vi "Measurement-DC.vi"(6 "引用句柄输出":refnum<file>, 7 "Ctl Refnum":refnum<vi>, 8 "error in (no error)":errorcluster caption="错误输入（无错误）", 9 "升温速率":dbl, 10 "结束温度":dbl, 11 "簇":T1) -> (0 "error out":errorcluster caption="错误输出", 1 "极化电流":dbl, 2 "布尔":bool, 3 "当前温度":dbl)   [LabVIEW 2017]
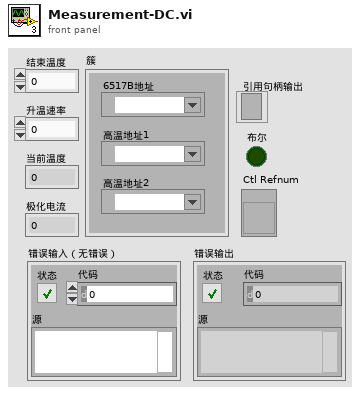
[diagram p1: front panel]
types:
  T1 = cluster{"6517B地址":refnum<visa-resource-name>, "高温地址1":refnum<visa-resource-name>, "高温地址2":refnum<visa-resource-name>}
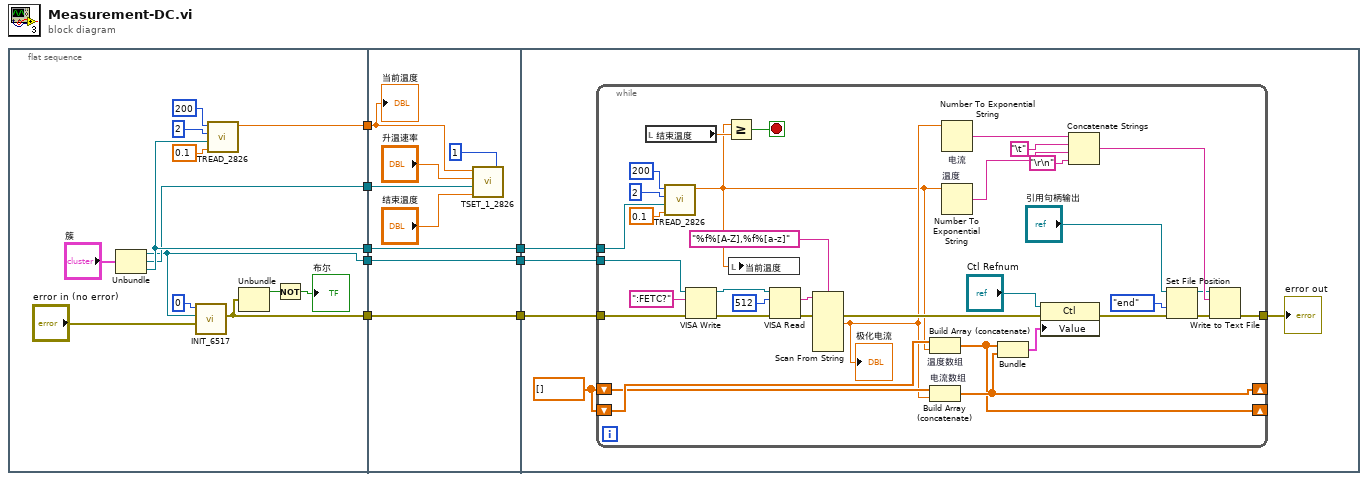
[diagram p0: block diagram]
diagram:
  n1 = flat-sequence {
    tunnel: [w17] -> w8
    tunnel: [w15] -> w6
    tunnel: [w14] -> w5
    tunnel: [w12] -> w3
    tunnel: [w11] -> w1
    tunnel: w8 -> [w29]
    tunnel: [w29] -> w7
    tunnel: w6 -> [w28]
    tunnel: w5 -> [w26]
    tunnel: [w23] -> w4
    tunnel: w3 -> [w23]
    tunnel: [w22] -> w2
    tunnel: w1 -> [w22]
    tunnel: w7 -> [w34]
    tunnel: w4 -> [w33]
    tunnel: w2 -> [w32]
    frame #0 {
      n2 = Unbundle("簇") -> ("6517B地址"=w12:refnum<visa-resource-name>, "高温地址1"=w15:refnum<visa-resource-name>, "高温地址2"=w17:refnum<visa-resource-name>)
      n3 = call "INIT_6517.vi"("error in (no error)"="error in (no error)", "VISA resource name"=w12, "Vin"=0) -> ("error out"=w11:errorcluster)  [unwired: 7 in, 1 out]
      n4 = call "TREAD_2826.vi"("Unknown Param 2"=0.1, "VISA resource name"=w17, "Address No."=2, "Unknown Param"=200) -> ("PV"=w14:dbl)  [unwired: 3 out]
      n5 = Unbundle(w11) -> ("status"=w9:bool)  [unwired: 2 out]
      n6 = Not(x=w9) -> (.not. x?=→"布尔":bool)
    }
    frame #1 {
      n7 = call "TSET_1_2826.vi"("Address No."=1, "T-Ending, C"="结束温度", "VISA resource name"=w28, "cooling/heating rate, C/min"="升温速率", "T-Starting, C"=w26) -> ()
      "当前温度" <- w26
    }
    frame #2 {
      w31 = dbl[] []
      n8 = while {
        tunnel: w34 -> [w69]
        tunnel: w33 -> [w62]
        tunnel: w32 -> [w61]
        shift-right: [w51] -> _
        shift-left: w31 -> [w54]
        shift-right: [w52] -> _
        shift-left: w31 -> [w53]
        tunnel: [w46] -> w30
        stop <- w64 stop-if-true
        n9 = local read "结束温度"() -> (w65:dbl)
        n10 = call "TREAD_2826.vi"("Unknown Param 2"=0.1, "VISA resource name"=w69, "Address No."=2, "Unknown Param"=200) -> ("PV"=w35:dbl)  [unwired: 3 out]
        n11 = VISA Write(VISA resource name=w62, write buffer=":FETC?" ("写入缓冲区"), error in (no error)=w61) -> (VISA resource name out=w58:refnum<visa-resource-name>, error out=w60:errorcluster)  [unwired: 1 out]
        n12 = Greater Or Equal?(x=w35, y=w65) -> (x >= y?=w64:bool)
        n13 = local write "当前温度"(w35) -> ()
        n14 = VISA Read(VISA resource name=w58, byte count=u32 512 ("字节总数"), error in (no error)=w60) -> (read buffer=w57:string, error out=w56:errorcluster)  [unwired: 2 out]
        n15 = Scan From String(format string="%f%[A-Z],%f%[a-z]" ("格式字符串"), input string=w57, error in=w56) -> (error out=w48:errorcluster, output 1=w36:dbl)  [unwired: 1 in, 9 out]
        "极化电流" <- w36
        n16 = Build Array (concatenate) "温度数组"(w54, w35) -> (w51:dbl[])
        n17 = Build Array (concatenate) "电流数组"(w53, w36) -> (w52:dbl[])
        n18 = Number To Exponential String "电流"(number=w36) -> (E-format string=w43:string)  [unwired: 1 in, 2 out]
        n19 = Number To Exponential String "温度"(number=w35) -> (E-format string=w42:string)  [unwired: 3 out]
        n20 = Bundle(w51, w52) -> (w49:cluster{dbl[], dbl[]})  [unwired: 1 in]
        n21 = property class="Ctl"(reference="Ctl Refnum", error in=w48, "Value"=w49) -> (error out=w45:errorcluster)  [unwired: 1 out]
        n22 = Concatenate Strings(w43, "\t", w42, "\r\n") -> (w39:string)
        n23 = Set File Position(refnum="引用句柄输出", from (0:start)=enum16{"start", "end", "current"}."end" ("自（0:起始）"), error in=w45) -> (refnum out=w38:refnum<file>, error out=w47:errorcluster)  [unwired: 1 out]
        n24 = Write to Text File(file (use dialog)=w38, text=w39, error in=w47) -> (error out=w46:errorcluster)  [unwired: 1 in, 2 out]
      }
      "error out" <- w30
    }
  }
